vi "TEST_bench_HM_times_x_preload_N22.vi"() -> ()   [LabVIEW 2017]
uses:
  fixed-point/typeDefs/x_vec_type.ctl
  <vilib>/rvi/Memory/Memory_Emulation/nirvimemoryFastEmulation.vi
  <vilib>/rvi/Memory/Memory_Emulation/nirvimemoryEmulation.vi
  <vilib>/rvi/Emulation/niFpgaEmulationIsFPGAContextNoSignature.vi
  <vilib>/rvi/DataTransferAndStorage/Container/Common/niFpgaContainerGetUniqueNameForEmu.vi
  <vilib>/rvi/Emulation/niFpgaProcessEmulError.vi
  <vilib>/rvi/Emulation/niFpgaSctlEmulationGetInTimedLoop.vi
  <vilib>/rvi/errors/nirviReportUnexpectedCaseInternalError (U32).vi
  <vilib>/rvi/DataTransferAndStorage/Container/XNode/niFpgaContainer.xnode
panel:
  in  "x_vec":T1=[0.6000000238418579, 0.6000000238418579, -0.5999999940395355, -0.5999999940395355, 0.6000000238418579, 0.6000000238418579, 0.6000000238418579, 0.6000000238418579, -0.5999999940395355, 0.6000000238418579, -0.5999999940395355, -4.0, 0.0, 0.0, 0.0, 0.0, 0.0, 0.0, 0.0, 0.0, 0.0, 0.0, 0.0, 0.0, 0.0]
  in  "Ncol":u16
  in  "Ns":u16
  in  "nuN_mpc":u16
  in  "big_mat_data":fxp<+/-,32,3>[](array[numeric])=[0.0, 0.0, 0.0, 0.0, 0.0, 0.0, 0.0, 0.0, 0.0, 0.0, 0.0, 0.0]
  out "preload result":fxp<+/-,32,3>[](array[numeric]) format="%.31g"
  out "primary result":fxp<+/-,32,3>[](array[numeric]) format="%.31g"
  in  "primary_write_addr":u16
  in  "preload_vec":fxp<+/-,32,3>[](array[numeric])=[0.0, 0.0, 0.0, 0.0, 0.0, 0.0, 0.0, 0.0, 0.0, 0.0, 0.0, 0.0]
  in  "preload_addr":u16
  in  "StartIndex":u16
  out "A*x":fxp<+/-,32,3>[](array[numeric])
  in  "SLMAX":fxp<+/-,18,5>
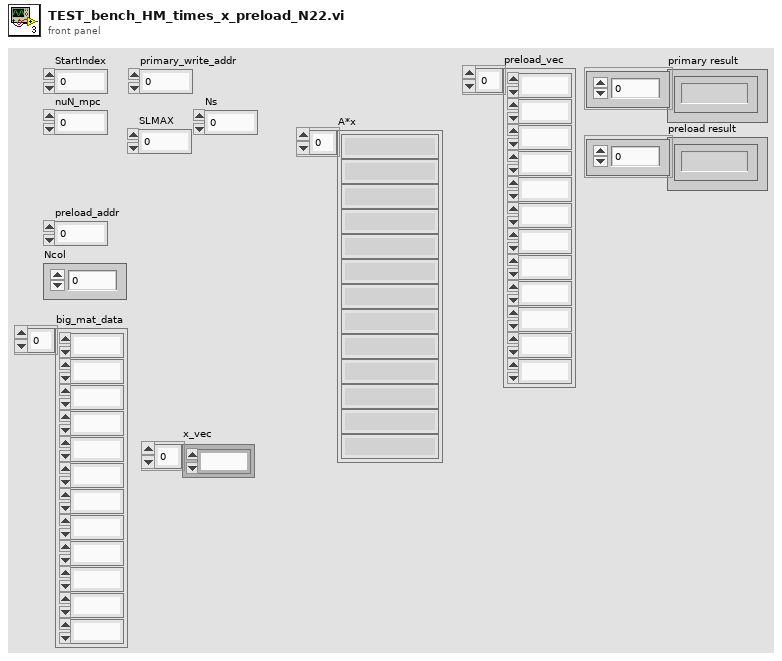
[diagram p1: front panel]
types:
  T1 = typedef "x_vec_type.ctl" = fxp<+/-,32,6>[]
  T2 = typedef "ziyi_pipe_N22.ctl" = T3[]
  T3 = typedef "x_qp_scalar.ctl" = fxp<+/-,32,6>
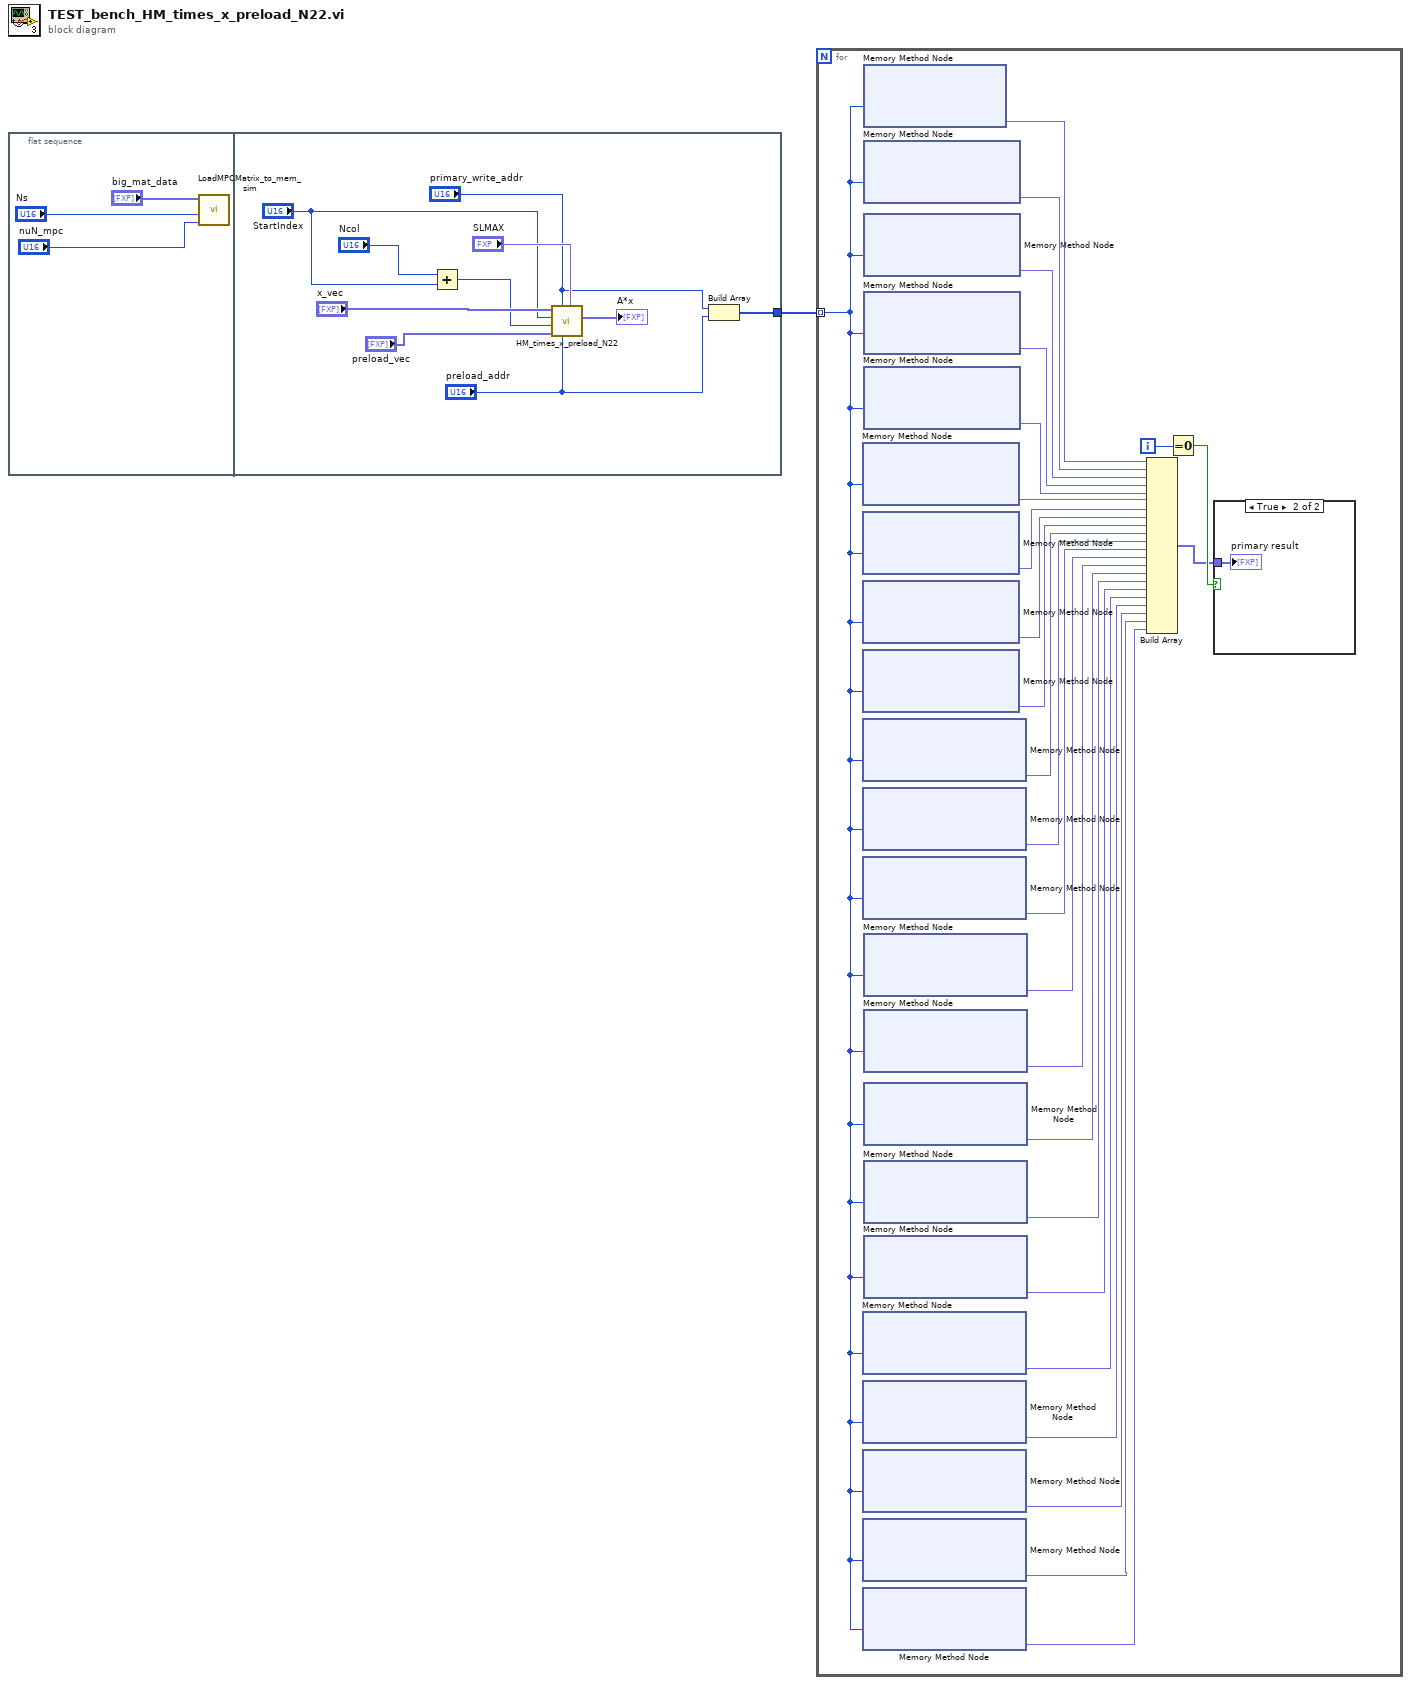
[diagram p0: block diagram]
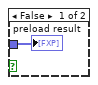
[diagram p2: hidden frame]
diagram:
  n1 = flat-sequence {
    tunnel: [w14] -> w1
    frame #0 {
      n2 = call "LoadMPCMatrix_to_mem_sim.vi"("nuN_mpc"="nuN_mpc", "Ns"="Ns", "big_mat_data"="big_mat_data") -> ()  [unwired: 9 in]
    }
    frame #1 {
      n3 = Add(x="Ncol", y="StartIndex") -> (x+y=w5:u16)
      n4 = call "HM_times_x_preload_N22.vi"("SLMAX"="SLMAX", "preload_addr"="preload_addr", "primary_write_addr"="primary_write_addr", "preload_vec"="preload_vec", "Ns+StartIndex"=w5, "StartIndex"="StartIndex", "x_vec"="x_vec") -> ("A*x"=→"A*x":T2)  [unwired: 3 in, 1 out]
      n5 = Build Array("primary_write_addr", "preload_addr") -> (w14:u16[])
    }
  }
  n6 = for {
    tunnel: w1 -> [w16] mode=indexing
    i -> [w26]
    n7 = xnode ("Memory Method Node")("Address"=w16) -> ("Data"=w35:fxp<+/-,32,4>)  [unwired: 1 in, 1 out]
    n8 = xnode ("Memory Method Node")("Address"=w16) -> ("Data"=w34:fxp<+/-,32,4>)  [unwired: 1 in, 1 out]
    n9 = xnode ("Memory Method Node")("Address"=w16) -> ("Data"=w33:fxp<+/-,32,4>)  [unwired: 1 in, 1 out]
    n10 = xnode ("Memory Method Node")("Address"=w16) -> ("Data"=w32:fxp<+/-,32,4>)  [unwired: 1 in, 1 out]
    n11 = xnode ("Memory Method Node")("Address"=w16) -> ("Data"=w31:fxp<+/-,32,4>)  [unwired: 1 in, 1 out]
    n12 = xnode ("Memory Method Node")("Address"=w16) -> ("Data"=w30:fxp<+/-,32,4>)  [unwired: 1 in, 1 out]
    n13 = xnode ("Memory Method Node")("Address"=w16) -> ("Data"=w29:fxp<+/-,32,4>)  [unwired: 1 in, 1 out]
    n14 = xnode ("Memory Method Node")("Address"=w16) -> ("Data"=w20:fxp<+/-,32,4>)  [unwired: 1 in, 1 out]
    n15 = xnode ("Memory Method Node")("Address"=w16) -> ("Data"=w19:fxp<+/-,32,4>)  [unwired: 1 in, 1 out]
    n16 = xnode ("Memory Method Node")("Address"=w16) -> ("Data"=w18:fxp<+/-,32,4>)  [unwired: 1 in, 1 out]
    n17 = xnode ("Memory Method Node")("Address"=w16) -> ("Data"=w17:fxp<+/-,32,4>)  [unwired: 1 in, 1 out]
    n18 = xnode ("Memory Method Node")("Address"=w16) -> ("Data"=w15:fxp<+/-,32,4>)  [unwired: 1 in, 1 out]
    n19 = xnode ("Memory Method Node")("Address"=w16) -> ("Data"=w40:fxp<+/-,32,4>)  [unwired: 1 in, 1 out]
    n20 = xnode ("Memory Method Node")("Address"=w16) -> ("Data"=w39:fxp<+/-,32,4>)  [unwired: 1 in, 1 out]
    n21 = xnode ("Memory Method Node")("Address"=w16) -> ("Data"=w38:fxp<+/-,32,4>)  [unwired: 1 in, 1 out]
    n22 = xnode ("Memory Method Node")("Address"=w16) -> ("Data"=w37:fxp<+/-,32,4>)  [unwired: 1 in, 1 out]
    n23 = xnode ("Memory Method Node")("Address"=w16) -> ("Data"=w36:fxp<+/-,32,4>)  [unwired: 1 in, 1 out]
    n24 = xnode ("Memory Method Node")("Address"=w16) -> ("Data"=w25:fxp<+/-,32,4>)  [unwired: 1 in, 1 out]
    n25 = xnode ("Memory Method Node")("Address"=w16) -> ("Data"=w24:fxp<+/-,32,4>)  [unwired: 1 in, 1 out]
    n26 = xnode ("Memory Method Node")("Address"=w16) -> ("Data"=w23:fxp<+/-,32,4>)  [unwired: 1 in, 1 out]
    n27 = xnode ("Memory Method Node")("Address"=w16) -> ("Data"=w22:fxp<+/-,32,4>)  [unwired: 1 in, 1 out]
    n28 = xnode ("Memory Method Node")("Address"=w16) -> ("Data"=w21:fxp<+/-,32,4>)  [unwired: 1 in, 1 out]
    n29 = Build Array(w40, w39, w38, w37, w36, w35, w34, w33, w32, w31, w30, w29, w25, w24, w23, w22, w21, w20, w19, w18, w17, w15) -> (w27:fxp<+/-,32,4>[])
    n30 = Equal To 0?(x=w26) -> (x = 0?=w28:bool)
    n31 = case shown="True" w28 {
      tunnel: w27 -> [w41 w42]
      frame False {
        "preload result" <- w41
      }
      frame True {
        "primary result" <- w42
      }
    }
  }
